vi "SCCSup_Dynam 3ButtonDialog.vi"(6 "Right Button Text":string, 7 "Window Title":string, 8 "error in (no error)":errorcluster, 9 "Center Button Text":string, 10 "Left Button Text":string, 11 "message":string) -> (0 "error out":errorcluster, 3 "Which Button?":T1(ring))   [LabVIEW 2017]
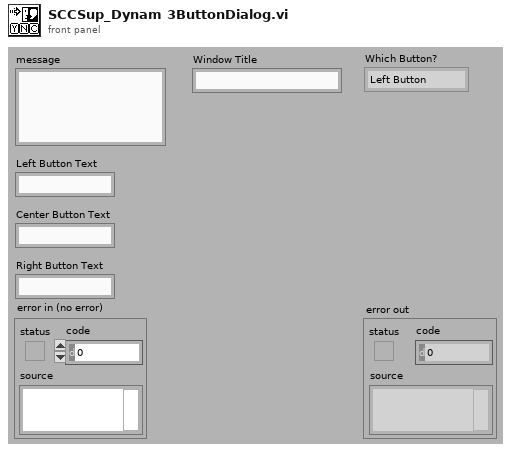
[diagram p1: front panel]
types:
  T1 = enum16{"Left Button", "Center Button", "Right Button", "Window Close"}
  T2 = cluster{"Left Button Key Shortcut":cluster{"Control":bool, "Shift":bool, "Key":string}, "Center Button Key Shortcut":cluster{"Control":bool, "Shift":bool, "Key":string}, "Right Button Key Shortcut":cluster{"Control":bool, "Shift":bool, "Key":string}}
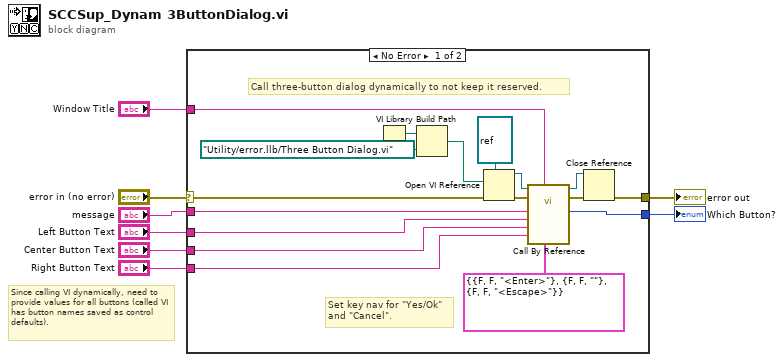
[diagram p0: block diagram]
diagram:
  # "Since calling VI dynamically, need to provide values for all buttons (called VI has button names saved as control defaults)."
  n1 = case shown="No Error" "error in (no error)" {
    selector: "error in (no error)" -> [w10 w26]
    tunnel: [w19 w26] -> w8
    tunnel: "Window Title" -> [w16 _]
    tunnel: "message" -> [w15 _]
    tunnel: [w14 _] -> w4
    tunnel: "Left Button Text" -> [w11 _]
    tunnel: "Center Button Text" -> [w12 _]
    tunnel: "Right Button Text" -> [w13 _]
    frame No Error {
      # "Set key nav for \"Yes/Ok\" and \"Cancel\"."
      # "Call three-button dialog dynamically to not keep it reserved."
      n2 = VI Library() -> (path=w25:path)
      n3 = Build Path(base path=w25, name or relative path=path "Utility/error.llb/Three Button Dialog.vi") -> (appended path=w23:path)
      n4 = Open VI Reference(type specifier VI Refnum (for type only)=refnum<vi> refnum, vi path=w23, error in (no error)=w10) -> (vi reference=w21:refnum<vi>, error out=w9:errorcluster)  [unwired: 3 in]
      n5 = call-by-ref "?"(reference=w21, error in=w9, "Keyboard Shortcuts (Left is <Enter>)"=T2 {"Left Button Key Shortcut"={"Control"=FALSE, "Shift"=FALSE, "Key"="<Enter>"}, "Center Button Key Shortcut"={"Control"=FALSE, "Shift"=FALSE, "Key"=""}, "Right Button Key Shortcut"={"Control"=FALSE, "Shift"=FALSE, "Key"="<Escape>"}}, "Window Title (\"\")"=w16, "Right Button Text (\"Cancel\")"=w13, "Center Button Text (\"No\")"=w12, "Left Button Text (\"Yes\")"=w11, "message"=w15) -> (reference out=w18:refnum<vi>, error out=w20:errorcluster, "Which Button?"=w14:T1)  [unwired: 5 in]
      n6 = Close Reference(reference=w18, error in (no error)=w20) -> (error out=w19:errorcluster)
    }
    frame Error {
    }
  }
  "error out" <- w8
  "Which Button?" <- w4
